vi "Format Block.vi"(4 "Data":string) -> (7 "Formatted Block":string)   [LabVIEW 2024, in "CTI.lvlib" / "VisaComms.lvclass"]
uses:
  VisaComms.lvclass
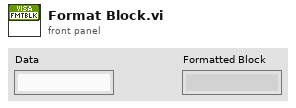
[diagram p1: front panel]
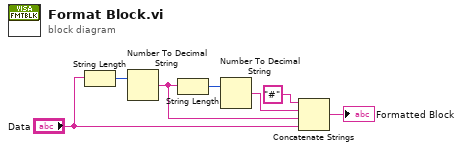
[diagram p0: block diagram]
diagram:
  n1 = String Length(string="Data") -> (length=w7:i32)
  n2 = Number To Decimal String(number=w7) -> (decimal integer string=w3:string)  [unwired: 1 in]
  n3 = String Length(string=w3) -> (length=w6:i32)
  n4 = Number To Decimal String(number=w6) -> (decimal integer string=w4:string)  [unwired: 1 in]
  n5 = Concatenate Strings("#" ("string"), w4, w3, "Data") -> (→"Formatted Block":string)
